vi "Get Port Parameters.vi"(8 "error in (no error)":errorcluster, 11 "niDTS Comm Serial in":refnum<class "niDTS Comm Serial.lvclass">) -> (0 "error out":errorcluster, 2 "Port Parameters":T1={"baud rate "=115200, "data bits"=8, "Enable Termination Char"=TRUE, "flow control"=0, "parity"=enum."None", "timeout (ms) "=5000, "stop bits"=10, "termination char"=10} {"termination char" format="%.0x"; "stop bits" items=["1.0"=10, "1.5"=15, "2.0"=20]; "flow control" items=["None", "XON/XOFF", "RTS/CTS", "XON/XOFF & RTS/CTS", "DTR/DSR", "XON/XOFF & DTR/DSR"]}, 3 "niDTS Comm Serial out":refnum<class "niDTS Comm Serial.lvclass">)   [LabVIEW 2015, in "niDTS CommLib.lvlib" / "niDTS Comm Serial.lvclass"]
uses:
  niDTS Comm Serial.lvclass
  niDTS Comm Serial.lvclass/niDTS Comm Serial.ctl
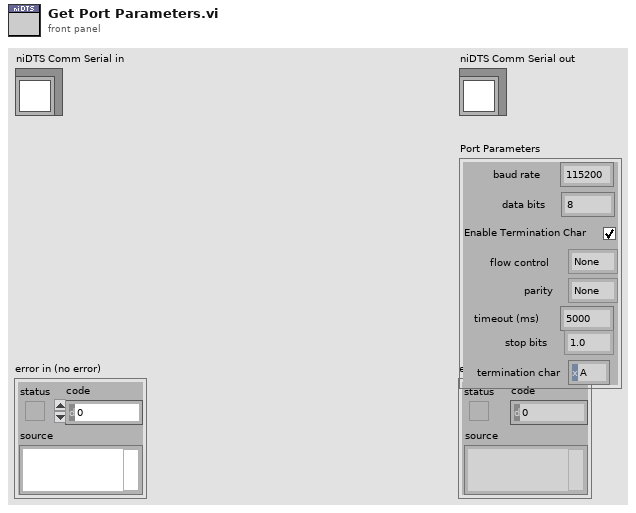
[diagram p1: front panel]
types:
  T1 = cluster{"baud rate ":u32, "data bits":u16, "Enable Termination Char":bool, "flow control":u16, "parity":enum16{"None", "Odd", "Even", "Mark", "Space"}, "timeout (ms) ":u32, "stop bits":u16, "termination char":u8}
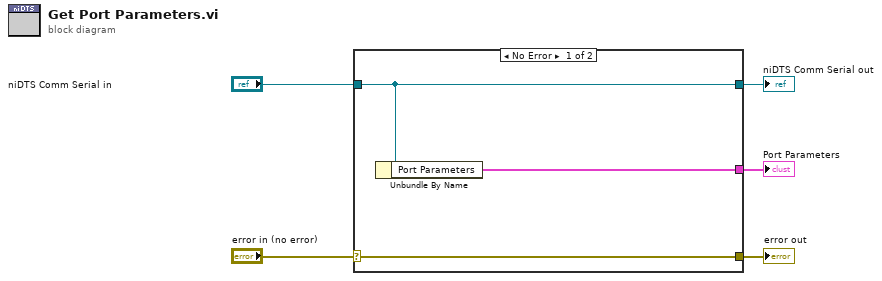
[diagram p0: block diagram]
diagram:
  n1 = case shown="No Error" "error in (no error)" {
    selector: "error in (no error)" -> [w8 w9]
    tunnel: [w8 w9] -> w4
    tunnel: [w7 w10] -> w2
    tunnel: "niDTS Comm Serial in" -> [w7 w10]
    tunnel: [w6 _] -> w1
    frame No Error {
      n2 = Unbundle By Name(w7) -> ("Port Parameters"=w6:T1)
    }
    frame Error {
    }
  }
  "error out" <- w4
  "niDTS Comm Serial out" <- w2
  "Port Parameters" <- w1
